vi "Initialize Attributes.vi"(8 "error in (no error)":errorcluster, 10 "Attribute Data":variant, 11 "CS++PVMonitor in":refnum<class "CS++PVMonitor.lvclass">) -> (0 "error out":errorcluster, 2 "Found?":bool, 3 "CS++PVMonitor out":refnum<class "CS++PVMonitor.lvclass">)   [LabVIEW 2013, in "CS++PVMonitor.lvlib" / "CS++PVMonitor.lvclass"]
doc: "Initialize object attribute.\n\nUnique resources should be allocated elsewhere!"
uses:
  CS++PVMonitor.lvclass
  CS++BaseActor/CS++BaseActor.lvclass
  CS++PVMonitor.lvclass/CS++PVMonitor.ctl
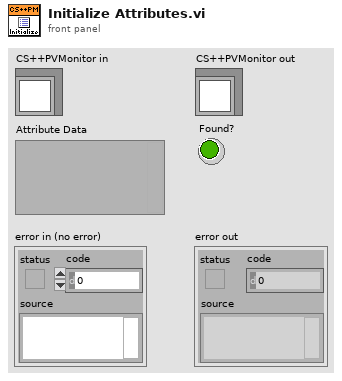
[diagram p1: front panel]
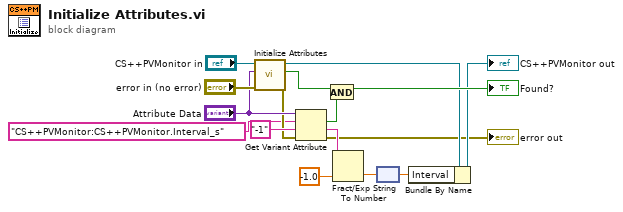
[diagram p0: block diagram]
diagram:
  n1 = call-parent "Initialize Attributes.vi"("error in (no error)"="error in (no error)", "Attribute Data"="Attribute Data", "CS++BaseActor in"="CS++PVMonitor in") -> ("error out"=w7:errorcluster, "Found?"=w16:bool, "CS++BaseActor out"=w3:refnum<class "CS++PVMonitor.lvclass">)  [unwired: 6 in]
  n2 = Get Variant Attribute(Variant="Attribute Data", name="CS++PVMonitor:CS++PVMonitor.Interval_s", default value (empty Variant)="-1", error in=w7) -> (found=w4:bool, value=w12:string, error out=→"error out":errorcluster)  [unwired: 1 out]
  n3 = And(x=w16, y=w4) -> (x .and. y?=→"Found?":bool)
  n4 = Fract/Exp String To Number(string=w12, default (0 dbl)=-1.0) -> (number=w10:dbl)  [unwired: 2 in, 1 out]
  n5 = node(w10) -> (w9:dbl[unit])
  n6 = Bundle By Name(cluster=w3, "Interval"=w9) -> (→"CS++PVMonitor out":refnum<class "CS++PVMonitor.lvclass">)
